vi "COMPORT-GetDeviceNamesOnCOMs.vi"(8 "error in (no error)":errorcluster) -> (0 "error out":errorcluster, 1 "#Resources":u32, 2 "COMs Arr":refnum<visa-resource-name>[](array[refnum]), 3 "COMDeviceList Arr":string[](array[string]))   [LabVIEW 2020, in "NOYITO 2 Channel Relay Driver.lvlib"]
uses:
  NOYITO 2 Channel Relay Driver.lvlib
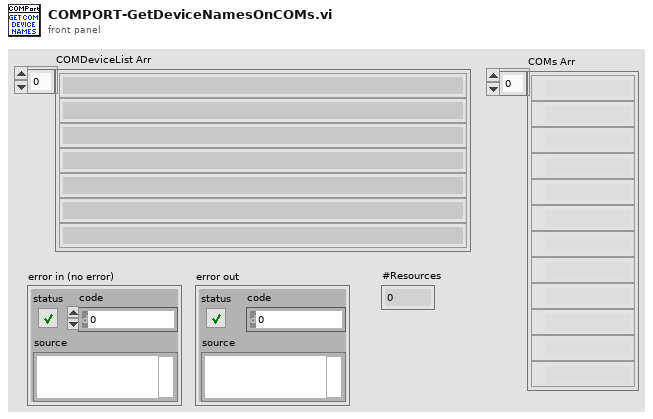
[diagram p1: front panel]
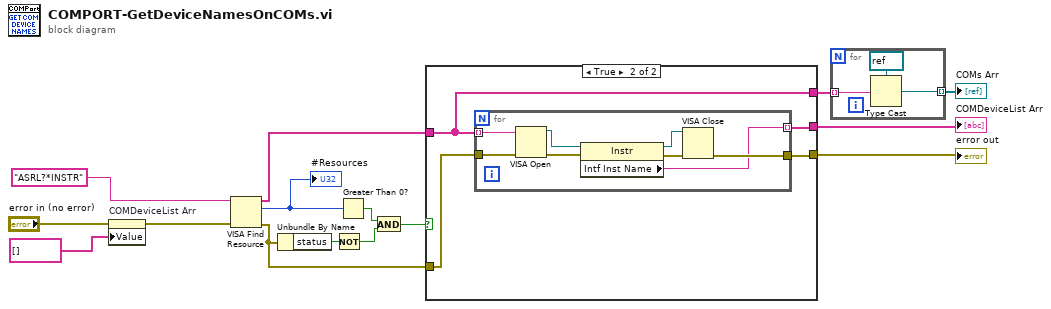
[diagram p0: block diagram]
diagram:
  n1 = property on="COMDeviceList Arr" class="Arr (strict)"(error in="error in (no error)", "Value"=string[] [] ("COMList")) -> (error out=w5:errorcluster)  [unwired: 1 in, 1 out]
  n2 = VISA Find Resource(8:w5, 11:"ASRL?*INSTR" ("expression (\"?*\")")) -> (0:w8:errorcluster, 2:w14:u32, 3:w9:string[])  [unwired: 1 in]
  "#Resources" <- w14
  n3 = Unbundle By Name(w8) -> ("status"=w13:bool)
  n4 = Not(x=w13) -> (.not. x?=w11:bool)
  n5 = Greater Than 0?(x=w14) -> (x > 0?=w10:bool)
  n6 = And(x=w10, y=w11) -> (x .and. y?=w12:bool)
  n7 = case shown="True" w12 {
    tunnel: w9 -> [_ w17]
    tunnel: w8 -> [w16 w20]
    tunnel: [w16 w19] -> w6
    tunnel: [_ w18] -> w7
    tunnel: [_ w17] -> w2
    frame False {
    }
    frame True {
      n8 = for {
        tunnel: w17 -> [w28] mode=indexing
        tunnel: [w23] -> w19
        tunnel: w20 -> [w22]
        tunnel: [w21] -> w18 mode=indexing
        n9 = VISA Open(error in (no error)=w22, VISA resource name=w28) -> (VISA resource name=w27:refnum<visa-resource-name>, error out=w26:errorcluster)  [unwired: 3 in]
        n10 = property class="Instr"(reference=w27, error in=w26) -> (reference out=w25:refnum<visa-resource-name>, error out=w24:errorcluster, "Intf Inst Name"=w21:string)
        n11 = VISA Close(VISA resource name=w25, error in (no error)=w24) -> (error out=w23:errorcluster)
      }
    }
  }
  "COMDeviceList Arr" <- w7
  "error out" <- w6
  n12 = for {
    tunnel: w2 -> [w31] mode=indexing
    tunnel: [w29] -> w1 mode=indexing
    n13 = Type Cast(type=refnum<visa-resource-name> refnum ("VISA resource name out"), x=w31) -> (*(type *) &x=w29:refnum<visa-resource-name>)
  }
  "COMs Arr" <- w1
